vi "Run dpinst for x86 or x64.vi"() -> ()   [LabVIEW 2011]
uses:
  <vilib>/Utility/sysdir.llb/System Directory Type.ctl
  OpenG.LIB/file/file.llb/Build Path - Traditional__ogtk.vi
  OpenG.LIB/file/file.llb/File Exists - Scalar__ogtk.vi
panel:
  out "error out":errorcluster
  # "Generic Driver Installation Tool\n\nDpinst.exe is a tool provided by Microsoft which, when placed in the same directory as a driver INF file, can be executed to automatically install drivers to the operating system.  \n\nThere are two different versions of this installer, one for 32-bit windows (x86) and another for 64-bit windows (x64).  We detect the windows version by searching for the  presence of the following directory on the system (one that would not exist on 32-bit systems):\n\nc:\\Windows\\SysWOW64\n\nParameters\nCommand Line parameters are passed directly to the dpinst.exe application"
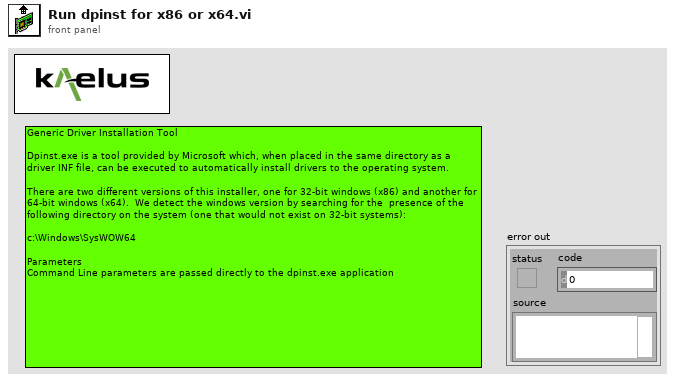
[diagram p1: front panel]
types:
  T1 = enum32{"invalid app kind", "Development System", "Run Time System", "Student Edition", "Embedded LabVIEW", "Evaluation", "Custom"}
  T2 = typedef "System Directory Type.ctl" = i32
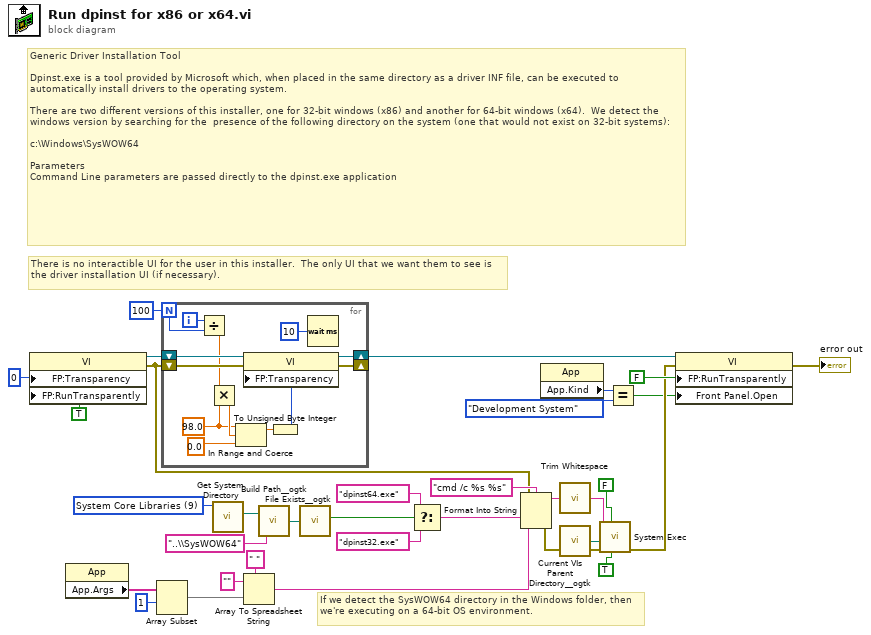
[diagram p0: block diagram]
diagram:
  w15 = T2 9 items=["User Home", "User Desktop", "User Documents", "User Application Data", "User Preferences", "User Temporary", "Public Documents", "Public Application Data", "Public Preferences", "System Core Libraries", "System Installed Libraries", "Application Files", "Boot Volume Root"] ("system directory type")
  # "Generic Driver Installation Tool\n\nDpinst.exe is a tool provided by Microsoft which, when placed in the same directory as a driver INF file, can be executed to automatically install drivers to the operating system.  \n\nThere are two different versions of this installer, one for 32-bit windows (x86) and another for 64-bit windows (x64).  We detect the windows version by searching for the  presence of the following directory on the system (one that would not exist on 32-bit systems):\n\nc:\\Windows\\SysWOW64\n\nParameters\nCommand Line parameters are passed directly to the dpinst.exe application"
  # "There is no interactible UI for the user in this installer.  The only UI that we want them to see is the driver installation UI (if necessary)."
  # "If we detect the SysWOW64 directory in the Windows folder, then we're executing on a 64-bit OS environment."
  n1 = property class="VI"("FP:Transparency"=u8 0, "FP:RunTransparently"=TRUE ("Front Panel Window:Run VI Transparently")) -> (reference out=w24:refnum<vi>, error out=w17:errorcluster)  [unwired: 2 in]
  n2 = property class="App"() -> ("App.Args"=w9:string[])  [unwired: 2 in, 2 out]
  n3 = Array Subset(array=w9, index=1) -> (w7:string[])  [unwired: 1 in]
  n4 = for {
    N: 100 -> [w41]
    shift-right: [w45] -> w23
    shift-left: w24 -> [w46]
    shift-right: [w44] -> _
    shift-left: w17 -> [w43]
    i -> [w42]
    w35 = 98.0
    n5 = Divide(x=w42, y=w41) -> (x/y=w40:dbl)
    n6 = Multiply(x=w40, y=w35) -> (x*y=w39:dbl)
    n7 = In Range and Coerce(upper limit=w35, x=w39, lower limit=0.0) -> (coerced(x)=w37:dbl)  [unwired: 1 out]
    n8 = To Unsigned Byte Integer(number=w37) -> (unsigned 8bit integer=w36:u8)
    n9 = property class="VI"(reference=w46, error in=w43, "FP:Transparency"=w36) -> (reference out=w45:refnum<vi>, error out=w44:errorcluster)
    n10 = Wait (ms)(milliseconds to wait=u32 10) -> ()  [unwired: 1 out]
  }
  n11 = call <vilib>:"Get System Directory.vi"("system directory type"=w15) -> ("system directory"=w14:path)  [unwired: 10 in]
  n12 = Array To Spreadsheet String(delimiter (Tab)=" ", array=w7, 3:"" ("format string")) -> (spreadsheet string=w4:string)
  n13 = call-poly "Build Path__ogtk.vi"("name or relative path"="..\\SysWOW64", "base path"=w14) -> ("appended path"=w12:path)
  n14 = call-poly "File Exists__ogtk.vi"("file path"=w12) -> ("is directory"=w11:bool)  [unwired: 6 in, 1 out]
  n15 = Select(t="dpinst64.exe" ("command"), s=w11, f="dpinst32.exe" ("command")) -> (s? t:f=w16:string)
  n16 = Format Into String(format string="cmd /c %s %s", error in=w17, w16, w4) -> (resulting string=w31:string, error out=w26:errorcluster)  [unwired: 1 in]
  n17 = property class="App"() -> ("App.Kind"=w3:T1)  [unwired: 2 in, 2 out]
  n18 = call <vilib>:"Trim Whitespace.vi"("string"=w31) -> ("trimmed string"=w10:string)  [unwired: 1 in]
  n19 = call "Current VIs Parent Directory__ogtk.vi"() -> ("Parent Directory (+ Relative)"=w33:path)  [unwired: 5 in]
  n20 = call <vilib>:"System Exec.vi"("run minimized? (F)"=TRUE, "wait until completion? (T)"=FALSE, "error in (no error)"=w26, "working directory"=w33, "command line"=w10) -> ("error out"=w19:errorcluster)  [unwired: 3 in, 3 out]
  n21 = Equal?(x=w3, y=T1."Development System" ("Application:Kind")) -> (x = y?=w1:bool)
  n22 = property class="VI"(reference=w23, error in=w19, "FP:RunTransparently"=FALSE ("Front Panel Window:Run VI Transparently"), "Front Panel.Open"=w1) -> (error out=→"error out":errorcluster)  [unwired: 1 out]
